vi "Enqueue Multi Msg.vi"(8 "error in":errorcluster, 9 "enable (T)":bool=TRUE, 11 "queue/message":string[](array[string])) -> (0 "error out":errorcluster)   [LabVIEW 2021]
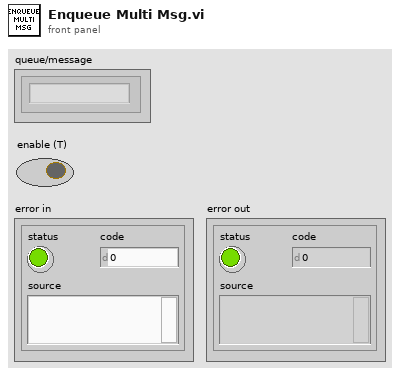
[diagram p1: front panel]
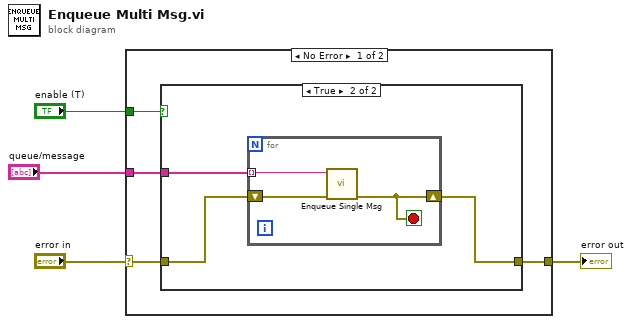
[diagram p0: block diagram]
diagram:
  n1 = case shown="No Error" "error in" {
    selector: "error in" -> [w6 w16]
    tunnel: "enable (T)" -> [w8 _]
    tunnel: "queue/message" -> [w7 _]
    tunnel: [w5 w16] -> w1
    frame No Error {
      n2 = case shown="True" w8 {
        tunnel: w7 -> [_ w12]
        tunnel: w6 -> [w9 w11]
        tunnel: [w9 w10] -> w5
        frame False {
        }
        frame True {
          n3 = for {
            tunnel: w12 -> [w15] mode=indexing
            shift-right: [w13] -> w10
            shift-left: w11 -> [w14]
            stop <- w13 stop-if-true
            n4 = call "Enqueue Single Msg.vi"("error in"=w14, "queue/message"=w15) -> ("error out"=w13:errorcluster)  [unwired: 9 in]
          }
        }
      }
    }
    frame Error {
    }
  }
  "error out" <- w1
